vi "Find_Pos(Index)_Particle_in_(X,Y)-1.vi"(2 "[X,Y] (n+1 Frame)":dbl[](array[numeric]), 3 "[X,Y] (n Frame)":dbl[](array[numeric]), 4 "Y2":dbl, 5 "X2":dbl, 6 "Y1":dbl, 7 "X1":dbl) -> (0 "Index in (n+1) Frame":i32, 1 "Index in (n) Frame":i32)   [LabVIEW 2017]
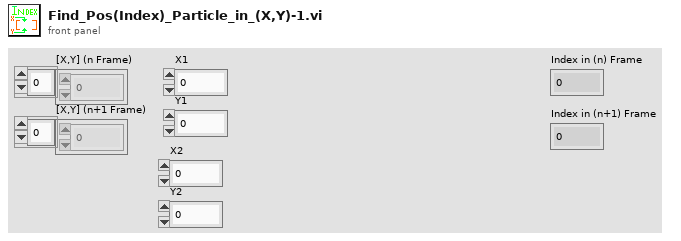
[diagram p1: front panel]
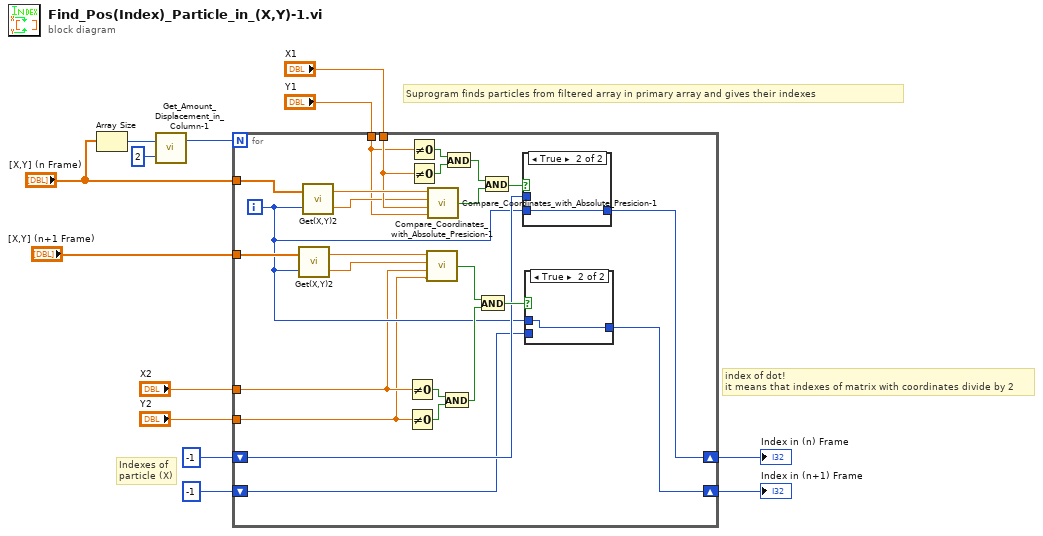
[diagram p0: block diagram]
diagram:
  # "index of dot! \nit means that indexes of matrix with coordinates divide by 2"
  # "Suprogram finds particles from filtered array in primary array and gives their indexes"
  # "Indexes of \nparticle (X)"
  n1 = Array Size(array="[X,Y] (n Frame)") -> (size(s)=w3:i32)
  n2 = call "Get_Amount_Displacement_in_Column-1.vi"("multiplier"=2 ("y"), "# Rows"=w3) -> ("Displ amount"=w1:i32)  [unwired: 1 out]
  n3 = for {
    N: w1 -> [_]
    tunnel: "[X,Y] (n Frame)" -> [w26]
    tunnel: "[X,Y] (n+1 Frame)" -> [w25]
    shift-right: [w28] -> w4
    shift-left: -1 -> [w27]
    shift-right: [w29] -> w5
    shift-left: -1 -> [w30]
    tunnel: "X2" -> [w17]
    tunnel: "Y2" -> [w16]
    tunnel: "X1" -> [w22]
    tunnel: "Y1" -> [w20]
    i -> [w24]
    n4 = call "Get(X,Y)2.vi"("[IN] index of (X,Y)"=w24, "[IN] Array coordi\nnates (X,Y) in Frame"=w25) -> ("[OUT] Y"=w15:dbl, "[OUT] X"=w18:dbl)
    n5 = call "Get(X,Y)2.vi"("[IN] index of (X,Y)"=w24, "[IN] Array coordi\nnates (X,Y) in Frame"=w26) -> ("[OUT] Y"=w21:dbl, "[OUT] X"=w23:dbl)
    n6 = Not Equal To 0?(x=w17) -> (x != 0?=w34:bool)
    n7 = Not Equal To 0?(x=w16) -> (x != 0?=w33:bool)
    n8 = Not Equal To 0?(x=w20) -> (x != 0?=w38:bool)
    n9 = Not Equal To 0?(x=w22) -> (x != 0?=w37:bool)
    n10 = call "Compare_Coordinates_with_Absolute_Presicion-1.vi"("X 1"=w18, "Y 1"=w15, "X 2"=w17, "Y 2"=w16) -> ("[OUT] Same coordinates?"=w14:bool)  [unwired: 1 in]
    n11 = call "Compare_Coordinates_with_Absolute_Presicion-1.vi"("X 1"=w23, "Y 1"=w21, "X 2"=w22, "Y 2"=w20) -> ("[OUT] Same coordinates?"=w19:bool)  [unwired: 1 in]
    n12 = And(x=w34, y=w33) -> (x .and. y?=w32:bool)
    n13 = And(x=w38, y=w37) -> (x .and. y?=w36:bool)
    n14 = And(x=w14, y=w32) -> (x .and. y?=w31:bool)
    n15 = And(x=w36, y=w19) -> (x .and. y?=w35:bool)
    n16 = case shown="True" w35 {
      tunnel: w30 -> [w41 _]
      tunnel: w24 -> [_ w42]
      tunnel: [w41 w42] -> w29
      frame False {
      }
      frame True {
      }
    }
    n17 = case shown="True" w31 {
      tunnel: w24 -> [_ w40]
      tunnel: [w39 w40] -> w28
      tunnel: w27 -> [w39 _]
      frame False {
      }
      frame True {
      }
    }
  }
  "Index in (n) Frame" <- w5
  "Index in (n+1) Frame" <- w4
